vi "Main.vi"() -> ()   [LabVIEW 2012]
uses:
  Consumer Message.ctl
  <vilib>/Utility/error.llb/Error Cluster From Error Code.vi
  <vilib>/ErrorRing/Error Ring.xnode
panel:
  in  "生产者错误":bool
  in  "消费者错误":bool
  out "消费者关闭？":bool
  out "待执行状态":string
  out "高优先级？":bool
  out "积压空间":u8(slide) scale=0.0..100.0
  out "已处理值":i32
  in  "高优先级消息":bool
  in  "标准优先级消息":bool
  in  "停止":bool
  # "待入队处理的\n消息数量"
  # "消费者循环中\n当前正在处理的数据"
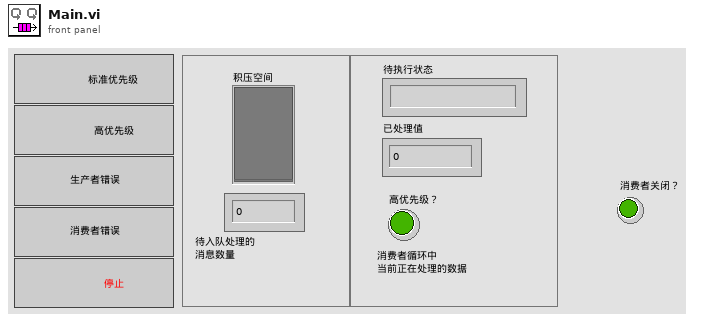
[diagram p1: front panel]
types:
  T1 = typedef "Consumer Message.ctl" = cluster{"消费者状态":string, "布尔数据":bool, "数值数据":i32, "错误":cluster{"状态":bool, "代码":i32, "源":string}}
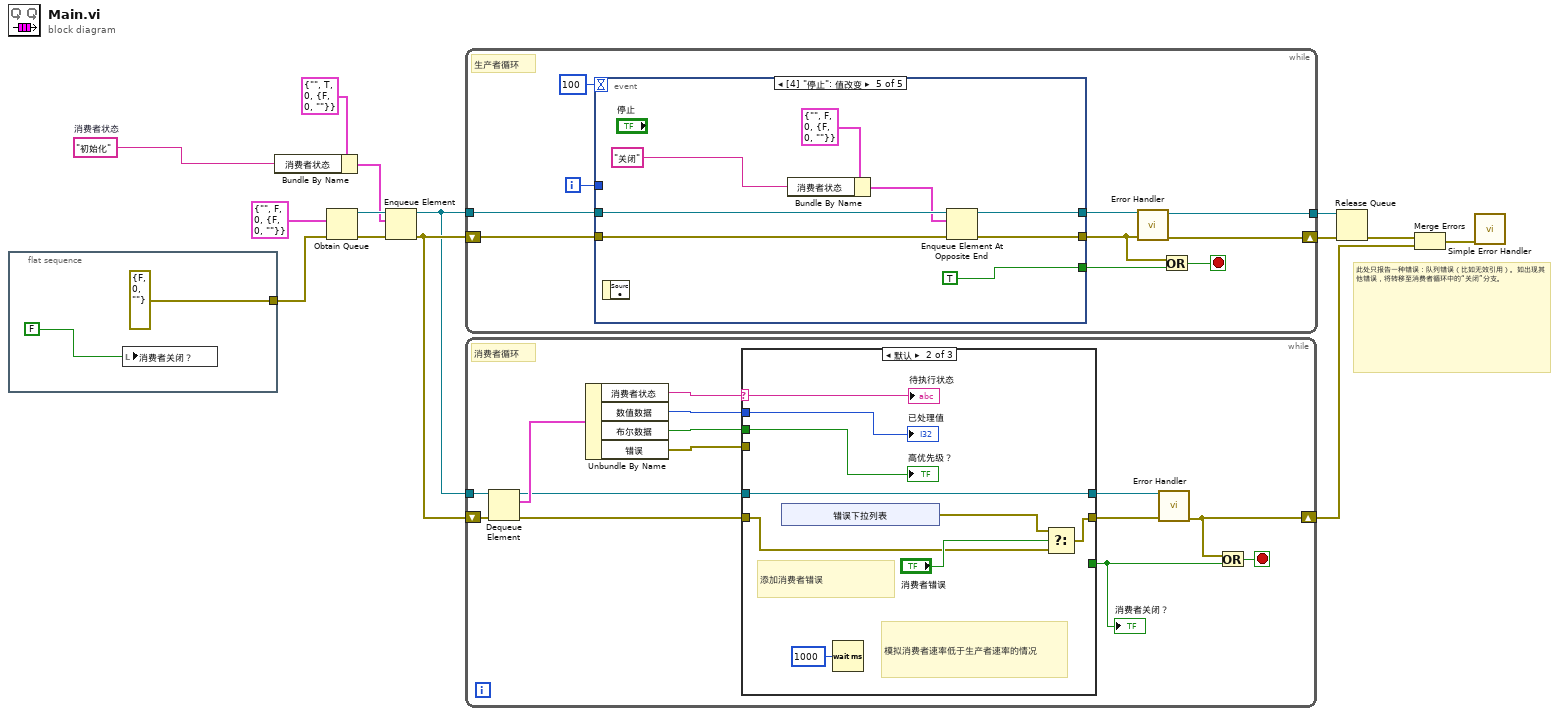
[diagram p0: block diagram]
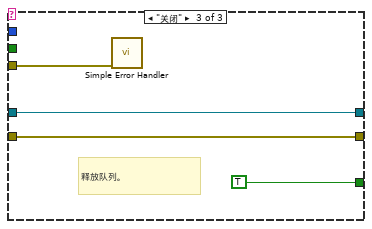
[diagram p3: hidden frame]
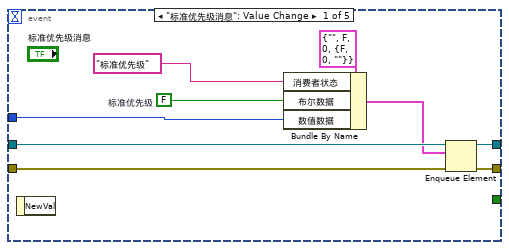
[diagram p4: hidden frame]
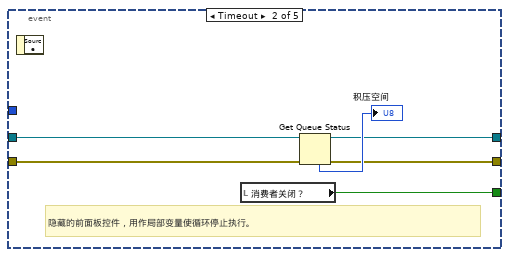
[diagram p5: hidden frame]
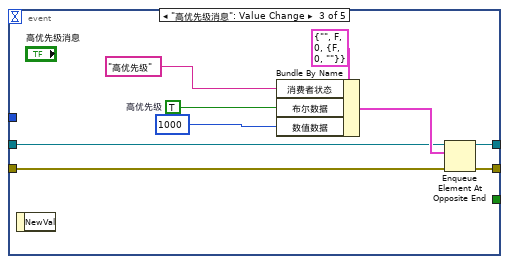
[diagram p6: hidden frame]
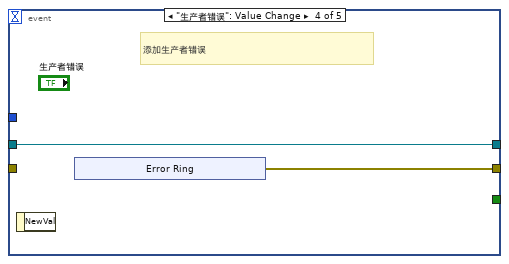
[diagram p7: hidden frame]
diagram:
  w6 = "初始化"  # 消费者状态
  # "此处只报告一种错误：队列错误（比如无效引用）。如出现其他错误，将转移至消费者循环中的“关闭”分支。"
  n1 = flat-sequence {
    tunnel: [cluster{"状态":bool, "代码":i32, "源":string} {"状态"=FALSE, "代码"=0, "源"=""} ("错误输入（无错误）")] -> w9
    frame #0 {
      n2 = local write "消费者关闭？"(FALSE ("停止循环（局部）")) -> ()
    }
  }
  n3 = Bundle By Name ("按名称捆绑")(cluster=T1 {"消费者状态"="", "布尔数据"=TRUE, "数值数据"=0, "错误"={"状态"=FALSE, "代码"=0, "源"=""}} ("消费者消息"), "消费者状态"=w6) -> (w7:T1)
  n4 = Obtain Queue ("获取队列引用")(element data type=T1 {"消费者状态"="", "布尔数据"=FALSE, "数值数据"=0, "错误"={"状态"=FALSE, "代码"=0, "源"=""}}, error in (no error)=w9) -> (queue out=w11:refnum<queue>, error out=w14:errorcluster)  [unwired: 3 in, 1 out]
  n5 = Enqueue Element ("元素入队列")(queue=w11, element=w7, error in (no error)=w14) -> (queue out=w10:refnum<queue>, error out=w12:errorcluster)  [unwired: 1 in, 1 out]
  n6 = while {
    tunnel: w10 -> [w26]
    shift-right: [w18] -> w4
    shift-left: w12 -> [w25]
    tunnel: [w17] -> w3
    i -> [w24]
    stop <- w20 stop-if-true
    # "生产者循环"
    n7 = event shown="[4] \"停止\": 值改变" {
      selector: _ -> [_ _ _ _ _]
      dyn-events: _ -> [_ _ _ _ _]
      timeout: 100 -> [_ _ _ _ _]
      tunnel: w26 -> [w35 w39 w42 w51 w64]
      tunnel: w25 -> [w33 w38 w49 _ w62]
      tunnel: [w34 w37 w50 w52 w61] -> w19
      tunnel: [_ w41 _ _ TRUE] -> w21
      tunnel: w24 -> [w32 _ _ _ _]
      tunnel: [w28 w36 w45 w51 w60] -> w23
      event "标准优先级消息": Value Change {
        w29 = FALSE  # 标准优先级
        n8 = event-data ("事件数据节点")() -> ()  [unwired: 1 in, 1 out]
        n9 = Bundle By Name ("按名称捆绑")(cluster=T1 {"消费者状态"="", "布尔数据"=FALSE, "数值数据"=0, "错误"={"状态"=FALSE, "代码"=0, "源"=""}}, "消费者状态"="标准优先级" ("字符串数据"), "布尔数据"=w29, "数值数据"=w32) -> (w31:T1)
        n10 = Enqueue Element ("元素入队列")(queue=w35, element=w31, error in (no error)=w33) -> (queue out=w28:refnum<queue>, error out=w34:errorcluster)  [unwired: 1 in, 1 out]
      }
      event Timeout {
        # "隐藏的前面板控件，用作局部变量使循环停止执行。"
        n11 = event-data ("事件数据节点")() -> ()  [unwired: 1 in, 1 out]
        n12 = local read "消费者关闭？"() -> (w41:bool)
        n13 = Get Queue Status ("获取队列状态")(queue=w39, error in (no error)=w38) -> (queue out=w36:refnum<queue>, error out=w37:errorcluster, # elements in queue=→"积压空间":i32)  [unwired: 1 in, 5 out]
      }
      event "高优先级消息": Value Change {
        w44 = TRUE  # 高优先级
        n14 = event-data ("事件数据节点")() -> ()  [unwired: 1 in, 1 out]
        n15 = Bundle By Name ("按名称捆绑")(cluster=T1 {"消费者状态"="", "布尔数据"=FALSE, "数值数据"=0, "错误"={"状态"=FALSE, "代码"=0, "源"=""}}, "消费者状态"="高优先级" ("字符串数据"), "布尔数据"=w44, "数值数据"=1000) -> (w47:T1)
        n16 = Enqueue Element At Opposite End ("队列最前端插入元素")(queue=w42, element=w47, error in (no error)=w49) -> (queue out=w45:refnum<queue>, error out=w50:errorcluster)  [unwired: 1 in, 1 out]
      }
      event "生产者错误": Value Change {
        # "添加生产者错误"
        n17 = event-data ("事件数据节点")() -> ()  [unwired: 1 in, 1 out]
        n18 = xnode "Error Ring"() -> ("错误输出"=w52:errorcluster)
      }
      event "停止": Value Change {
        n19 = event-data ("事件数据节点")() -> ()  [unwired: 1 in, 1 out]
        n20 = Bundle By Name ("按名称捆绑")(cluster=T1 {"消费者状态"="", "布尔数据"=FALSE, "数值数据"=0, "错误"={"状态"=FALSE, "代码"=0, "源"=""}}, "消费者状态"="关闭") -> (w57:T1)
        n21 = Enqueue Element At Opposite End ("队列最前端插入元素")(queue=w64, element=w57, error in (no error)=w62) -> (queue out=w60:refnum<queue>, error out=w61:errorcluster)  [unwired: 1 in, 1 out]
      }
    }
    n22 = call "Error Handler.vi"("错误输入"=w19, "队列输入"=w23) -> ("错误输出"=w18:cluster{"状态":bool, "代码":i32, "源":string}, "队列输出"=w17:refnum<queue>)  [unwired: 8 in]
    n23 = Or ("或")(x=w19, y=w21) -> (x .or. y?=w20:bool)
  }
  n24 = while {
    tunnel: w10 -> [w78]
    shift-right: [w67] -> w1
    shift-left: w12 -> [w77]
    stop <- w68 stop-if-true
    # "消费者循环"
    n25 = Dequeue Element ("元素出队列")(queue=w78, error in (no error)=w77) -> (queue out=w66:refnum<queue>, element=w76:T1, error out=w65:errorcluster)  [unwired: 1 in, 1 out]
    n26 = Unbundle By Name ("按名称解除捆绑")(w76) -> ("消费者状态"=w75:string, "数值数据"=w74:i32, "布尔数据"=w73:bool, "错误"=w70:cluster{"状态":bool, "代码":i32, "源":string})
    n27 = case shown="默认" w75 {
      selector: w75 -> [_ w86 _]
      tunnel: [_ _ TRUE] -> w69
      tunnel: w65 -> [w79 w82 w95]
      tunnel: [w79 w83 w95] -> w72
      tunnel: w74 -> [_ w89 _]
      tunnel: w73 -> [_ w88 _]
      tunnel: w66 -> [w80 w87 w96]
      tunnel: [w80 w87 w96] -> w71
      tunnel: w70 -> [_ _ w97]
      frame "初始化" {
      }
      frame Default {
        # "添加消费者错误"
        # "模拟消费者速率低于生产者速率的情况"
        n28 = xnode "错误下拉列表"() -> ("错误输出"=w81:errorcluster)
        n29 = Wait (ms) ("等待(ms)")(milliseconds to wait=u32 1000 ("等待时间（毫秒）")) -> ()  [unwired: 1 out]
        n30 = Select ("选择")(t=w81, s="消费者错误", f=w82) -> (s? t:f=w83:errorcluster)
        "已处理值" <- w89
        "高优先级？" <- w88
        "待执行状态" <- w86
      }
      frame "关闭" {
        # "释放队列。"
        n31 = call <vilib>:"Simple Error Handler.vi"("error in (no error)"=w97) -> ()  [unwired: 4 in, 5 out]
      }
    }
    "消费者关闭？" <- w69
    n32 = call "Error Handler.vi"("错误输入"=w72, "队列输入"=w71) -> ("错误输出"=w67:cluster{"状态":bool, "代码":i32, "源":string})  [unwired: 8 in, 1 out]
    n33 = Or ("或")(x=w67, y=w69) -> (x .or. y?=w68:bool)
  }
  n34 = Release Queue ("释放队列引用")(queue=w3, error in (no error)=w4) -> (error out=w2:errorcluster)  [unwired: 1 in, 2 out]
  n35 = Merge Errors ("合并错误")(w2, w1) -> (w5:errorcluster)
  n36 = call <vilib>:"Simple Error Handler.vi"("error in (no error)"=w5) -> ()  [unwired: 4 in, 5 out]
